vi "Create Load Reference VIs.vi"   [LabVIEW 2015]
types:
  T1 = typedef "ASC_UniqueIDStringParentIDStringName.ctl" = cluster{"Unique ID string":string, "Parent ID string":string, "Class Name (unlocalized)":string, "Class Name (localized)":string}
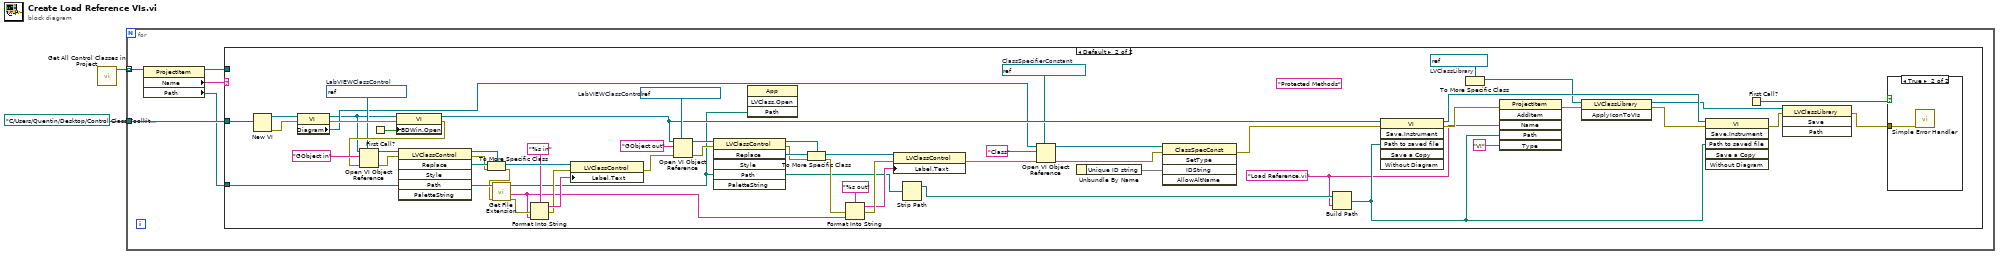
[diagram p0: block diagram]
diagram:
  n1 = call "Get All Control Classes in Project.vi"() -> ("All Control Classes"=w2:refnum<vi>[])  [unwired: 11 in]
  n2 = for {
    tunnel: w2 -> [w7] mode=indexing
    tunnel: path "C:/Users/Quentin/Desktop/Control Class Toolkit/Control Classes/GObject/Load Reference.vi" ("Path 2") -> [w4]
    n3 = property class="ProjectItem"(reference=w7) -> (reference out=w5:refnum<vi>, "Name"=w6:string, "Path"=w3:path)  [unwired: 1 in, 1 out]
    n4 = case shown="Default" w6 {
      tunnel: w5 -> [_ _]
      tunnel: w4 -> [_ w71]
      tunnel: w3 -> [_ w56]
      frame "GObject.lvclass", "Generic.lvclass" {
      }
      frame Default {
        w8 = "Protected Methods" ("Folder Name")
        w10 = refnum<vi> refnum  # LVClassLibrary
        w16 = "Load Reference.vi"
        w29 = refnum<vi> refnum  # ClassSpecifierConstant
        w32 = refnum<vi> refnum  # LabVIEWClassControl
        w67 = refnum<vi> refnum  # LabVIEWClassControl
        n5 = New VI(10:w71) -> (0:w62:errorcluster, 3:w70:refnum<vi>)  [unwired: 6 in]
        n6 = property class="VI"(reference=w70, error in=w62) -> (reference out=w22:refnum<vi>, error out=w61:errorcluster, "Diagram"=w30:refnum<vi>)
        n7 = First Call?() -> (First Call?: T/F=w34:bool)
        n8 = property class="VI"(reference=w22, error in=w61, "BDWin.Open"=w34) -> (reference out=w40:refnum<vi>, error out=w60:errorcluster)
        n9 = Open VI Object Reference(7:w32, 8:w60, 10:"GObject in" ("name/order"), 11:w22) -> (0:w63:errorcluster, 3:w68:refnum<vi>)
        n10 = invoke class="LVClassControl" method="Replace"(reference=w68, error in=w63, "Path"=w56) -> (reference out=w57:refnum<vi>, error out=w51:errorcluster, "Replace"=w59:refnum<vi>)  [unwired: 3 in, 3 out]
        n11 = To More Specific Class(target class=w57, reference=w59, error in=w51) -> (specific class reference=w58:refnum<vi>, error out=w50:errorcluster)
        n12 = call <vilib>:"Get File Extension.vi"("error in (no error)"=w50, "file"=w56) -> ("error out"=w49:errorcluster, "filename without extension"=w15:string, "dup file"=w39:path)  [unwired: 5 in, 2 out]
        n13 = Format Into String(format string="%s in", error in=w49, w15) -> (resulting string=w54:string, error out=w48:errorcluster)  [unwired: 1 in]
        n14 = property class="LVClassControl"(reference=w58, error in=w48, "Label.Text"=w54) -> (error out=w47:errorcluster)  [unwired: 1 out]
        n15 = Open VI Object Reference(7:w67, 8:w47, 10:"GObject out" ("name/order"), 11:w40) -> (0:w64:errorcluster, 3:w65:refnum<vi>)
        n16 = invoke class="LVClassControl" method="Replace"(reference=w65, error in=w64, "Path"=w39) -> (reference out=w52:refnum<vi>, error out=w46:errorcluster, "Replace"=w53:refnum<vi>)  [unwired: 3 in, 3 out]
        n17 = invoke class="App" method="LVClass.Open"("Path"=w39) -> ("LVClass.Open"=w13:refnum<vi>)  [unwired: 3 in, 3 out]
        n18 = To More Specific Class(target class=w52, reference=w53, error in=w46) -> (specific class reference=w43:refnum<vi>, error out=w45:errorcluster)
        n19 = Format Into String(format string="%s out", error in=w45, w15) -> (resulting string=w41:string, error out=w42:errorcluster)  [unwired: 1 in]
        n20 = property class="LVClassControl"(reference=w43, error in=w42, "Label.Text"=w41) -> (error out=w28:errorcluster)  [unwired: 1 out]
        n21 = Strip Path(path=w39) -> (stripped path=w38:path)  [unwired: 1 out]
        n22 = Open VI Object Reference(7:w29, 8:w28, 10:"Class" ("name/order"), 11:w30) -> (0:w26:errorcluster, 3:w27:refnum<vi>)
        n23 = Unbundle By Name() -> (w14:T1, "Unique ID string"=w21)
        n24 = invoke class="ClassSpecConst" method="SetType"(reference=w27, error in=w26, "IDString"=w21) -> (error out=w25:errorcluster)  [unwired: 2 in, 4 out]
        n25 = Build Path(base path=w38, name or relative path=w16) -> (appended path=w20:path)
        n26 = invoke class="VI" method="Save.Instrument"(reference=w40, error in=w25, "Path to saved file"=w20) -> (reference out=w23:refnum<vi>, error out=w37:errorcluster)  [unwired: 3 in, 4 out]
        n27 = To More Specific Class(target class=w10) -> (reference=w12:refnum<vi>, specific class reference=w11:refnum<vi>)  [unwired: 1 in, 1 out]
        n28 = invoke class="ProjectItem" method="AddItem"(error in=w37, "Name"=w16, "Path"=w20, "Type"="VI") -> (reference=w9:refnum<vi>, error out=w35:errorcluster)  [unwired: 1 in, 5 out]
        n29 = invoke class="LVClassLibrary" method="ApplyIconToVIs"(reference=w11, error in=w35) -> (reference out=w19:refnum<vi>, error out=w24:errorcluster)  [unwired: 1 in, 1 out]
        n30 = invoke class="VI" method="Save.Instrument"(reference=w23, error in=w24, "Path to saved file"=w20) -> (error out=w18:errorcluster)  [unwired: 3 in, 5 out]
        n31 = First Call?() -> (First Call?: T/F=w33:bool)
        n32 = invoke class="LVClassLibrary" method="Save"(reference=w19, error in=w18) -> (error out=w17:errorcluster)  [unwired: 2 in, 3 out]
        n33 = case shown="True" w33 {
          tunnel: w17 -> [_ w72]
          frame False {
          }
          frame True {
            n34 = call <vilib>:"Simple Error Handler.vi"("error in (no error)"=w72) -> ()  [unwired: 4 in, 5 out]
          }
        }
      }
    }
  }
